vi "rs3 create sensor.vi"(8 "error in (no error)":errorcluster, 10 "Sensor index":i32, 11 "Sensor list":u64) -> (0 "error out":errorcluster, 1 "Sensor out":u64, 2 "error":u64, 3 "Sensor list out":u64)   [LabVIEW 2017, in "libRealSense3.lvlib"]
doc: "Creates a SENSOR based on an input index to a SENSOR LIST.\n\nINPUT: \nSensor list Array of sensor handles\nIndex Input index \n\nOUTPUT:\nSensor out The SENSOR handle to be used for all subsequent communication\nError 0=no error"
uses:
  <vilib>/addons/RealSense/libRealSense3.lvlib
  Users/Greg McKaskle/Downloads/librealsense-1.12.1/librealsense-1.12.1/bin/Win32/realsense-d.dll
panel:
  # "RS3 Create Sensor"
  # "(C) 2017 Intel Corp.,  AGJ"
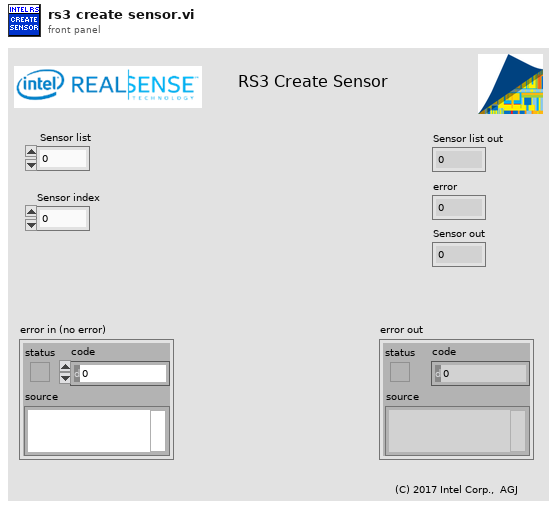
[diagram p1: front panel]
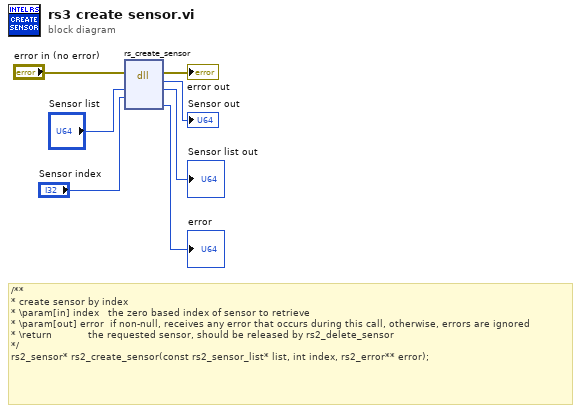
[diagram p0: block diagram]
diagram:
  # "/**\n* create sensor by index\n* \\param[in] index   the zero based index of sensor to retrieve\n* \\param[out] error  if non-null, receives any error that occurs during this call, otherwise, errors are ignored\n* \\return            the requested sensor, should be released by rs2_delete_sensor\n*/\nrs2_sensor* rs2_create_sensor(const rs2_sensor_list* list, int index, rs2_error** error);"
  n1 = dll-call lib="C:/Users/Greg McKaskle/Downloads/librealsense-1.12.1/librealsense-1.12.1/bin/Win32/realsense-d.dll" fn="rs_create_sensor"(error in="error in (no error)", "sensor list"="Sensor list", "index"="Sensor index") -> (error out=→"error out":errorcluster, "sensor"=→"Sensor out":u64, "sensor list"=→"Sensor list out":u64, "error"=→"error":u64)  [unwired: 4 in, 1 out]
